vi "Ocean Optics 2000 4000 Acquire Multiple Waveform.vi"() -> ()   [LabVIEW 2024]
doc: "Demonstrates measuring multiple spectra and displaying in a single waveform graph."
uses:
  Ocean Optics 2000 4000.lvlib
panel:
  in  "Delay Between Measurements (1 sec)":dbl=1.0
  in  "Number of Measurements (5)":i32=5
  out "Spectral Waveform":cluster{dbl[], dbl[]}[](graph)
  in  "Enable Strobe (Disabled)":bool
  in  "VISA resource name":refnum<visa-resource-name>
  # "(c) 2009-2016 National Instruments.  ALL RIGHTS RESERVED."
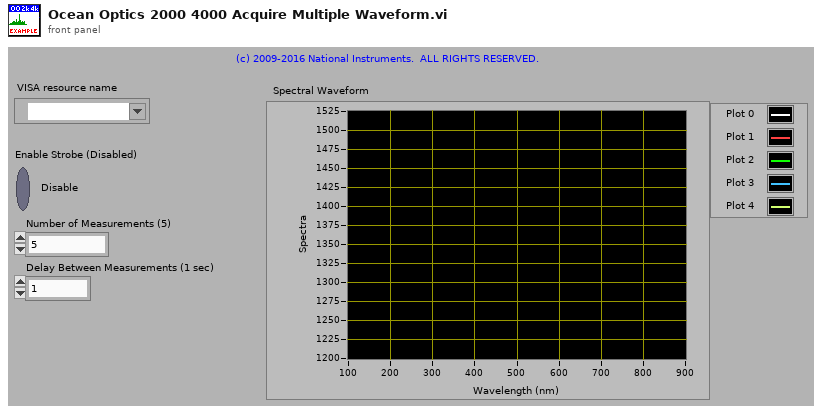
[diagram p1: front panel]
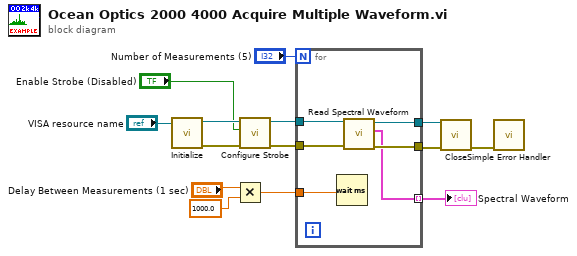
[diagram p0: block diagram]
diagram:
  n1 = call "Initialize.vi"("VISA resource name"="VISA resource name") -> ("error out"=w13:errorcluster, "VISA resource name out"=w14:refnum<visa-resource-name>)  [unwired: 2 in, 7 out]
  n2 = Multiply(x="Delay Between Measurements (1 sec)", y=1000.0) -> (x*y=w1:dbl)
  n3 = call "Configure Strobe.vi"("error in (no error)"=w13, "Enable Strobe (Disabled)"="Enable Strobe (Disabled)", "VISA resource name"=w14) -> ("error out"=w11:errorcluster, "VISA resource name out"=w12:refnum<visa-resource-name>)  [unwired: 7 out]
  n4 = for {
    N: "Number of Measurements (5)" -> [_]
    tunnel: w12 -> [w20]
    tunnel: w11 -> [w19]
    tunnel: [w18] -> w9
    tunnel: [w17] -> w8
    tunnel: [w16] -> w4 mode=indexing
    tunnel: w1 -> [w15]
    n5 = Wait (ms)(milliseconds to wait=w15) -> ()  [unwired: 1 out]
    n6 = call "Read Spectral Waveform.vi"("error in (no error)"=w19, "VISA resource name"=w20) -> ("error out"=w17:errorcluster, "Spectral Waveform"=w16:cluster{dbl[], dbl[]}, "VISA resource name out"=w18:refnum<visa-resource-name>)  [unwired: 7 out]
  }
  "Spectral Waveform" <- w4
  n7 = call "Close.vi"("error in (no error)"=w8, "VISA resource name"=w9) -> ("error out"=w7:errorcluster)  [unwired: 9 out]
  n8 = call <vilib>:"Simple Error Handler.vi"("error in (no error)"=w7) -> ()  [unwired: 1 in, 8 out]
